vi "No color_Stim Prot.vi"(8 "error in (no error)":errorcluster, 11 "Protocol Editor reference IN":refnum<vi>) -> (0 "error out":errorcluster, 3 "Protocol Editor reference OUT":refnum<vi>)   [LabVIEW 2012]
uses:
  <vilib>/Utility/miscctls.llb/LVRowAndColumnTypeDef.ctl
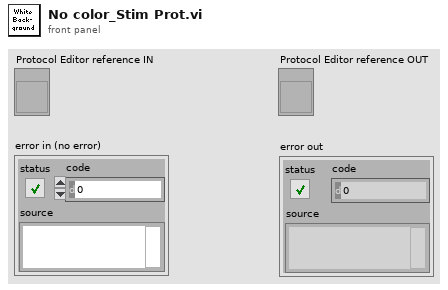
[diagram p1: front panel]
types:
  T1 = typedef "LVRowAndColumnTypeDef.ctl" = cluster{"Row":i32, "Column":i32}
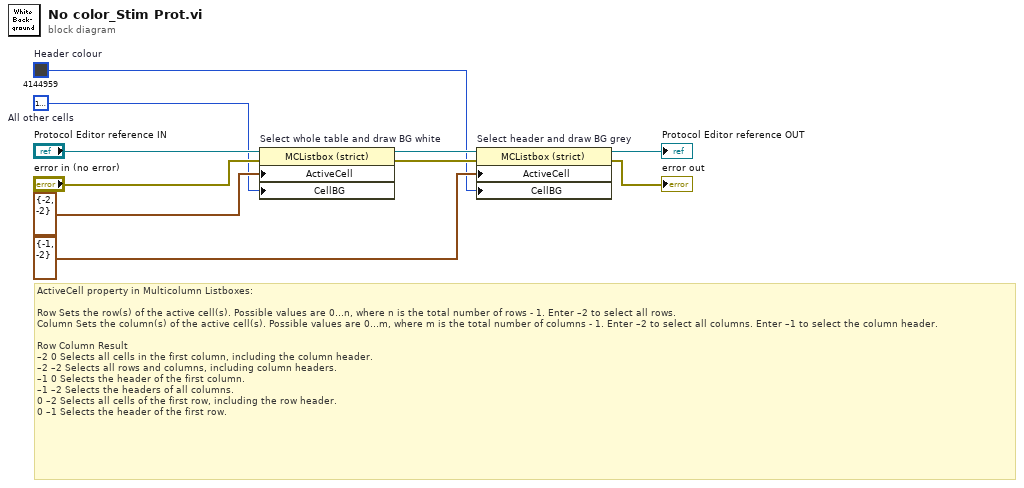
[diagram p0: block diagram]
diagram:
  w1 = u32 4144959  # Header colour
  w5 = u32 16777226  # All other cells
  # "ActiveCell property in Multicolumn Listboxes:\n\nRow Sets the row(s) of the active cell(s). Possible values are 0…n, where n is the total number of rows - 1. Enter –2 to select all rows. \nColumn Sets the column(s) of the active cell(s). Possible values are 0…m, where m is the total number of columns - 1. Enter –2 to select all columns. Enter –1 to select the column header. \n\nRow Column Result \n–2 0 Selects all cells in the first column, including the column header. \n–2 –2 Selects all rows and columns, including column headers. \n–1 0 Selects the header of the first column. \n–1 –2 Selects the headers of all columns. \n0 –2 Selects all cells of the first row, including the row header. \n0 –1 Selects the header of the first row."
  n1 = property on="Select whole table and draw BG white" class="MCListbox (strict)"(reference="Protocol Editor reference IN", error in="error in (no error)", "ActiveCell"=T1 {"Row"=-2, "Column"=-2} ("Active Cell:Active Cell"), "CellBG"=w5) -> (reference out=w4:refnum<vi>, error out=w3:errorcluster)
  n2 = property on="Select header and draw BG grey" class="MCListbox (strict)"(reference=w4, error in=w3, "ActiveCell"=T1 {"Row"=-1, "Column"=-2} ("Active Cell:Active Cell"), "CellBG"=w1) -> (reference out=→"Protocol Editor reference OUT":refnum<vi>, error out=→"error out":errorcluster)
